vi "Initialize.vi"(8 "error in (no error)":errorcluster, 9 "Reset? (T: Yes)":bool=TRUE, 10 "ID Query? (T: Yes)":bool=TRUE, 11 "VISA resource name":refnum<visa-resource-name>) -> (0 "error out":errorcluster, 3 "VISA resource name out":refnum<visa-resource-name>)   [LabVIEW 2022 SP3, in "Agilent ENA Series.lvlib"]
doc: "Establishes communication with the instrument and optionally performs an instrument identification query and/or an instrument reset. It also places the instrument in a default state needed for other instrument driver operations. Therefore, call this VI before calling other instrument driver VIs for this instrument. Generally, you need to call the <B>Initialize VI</B> only once at the beginning of an application.\n\n<b>Note:</b>\nE5080A model support enabled by configuring the Emulation Mode \nSystem -> System Setting -> Code Emulation -> 5071"
uses:
  Agilent ENA Series.lvlib
  <vilib>/regexp/Match Regular Expression.xnode
panel:
  # "(c) 2005-2021 National Instruments.  ALL RIGHTS RESERVED."
  # "Note:\nE5080A, E5080B model support enabled by configuring the Emulation Mode \nSystem -> System Setting -> Code Emulation -> 5071"
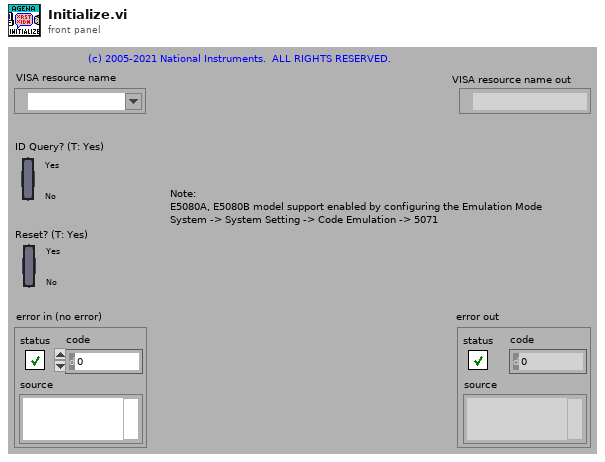
[diagram p1: front panel]
types:
  T1 = cluster{"Status":bool, "Code":i32, "Source (VI Name)":string}
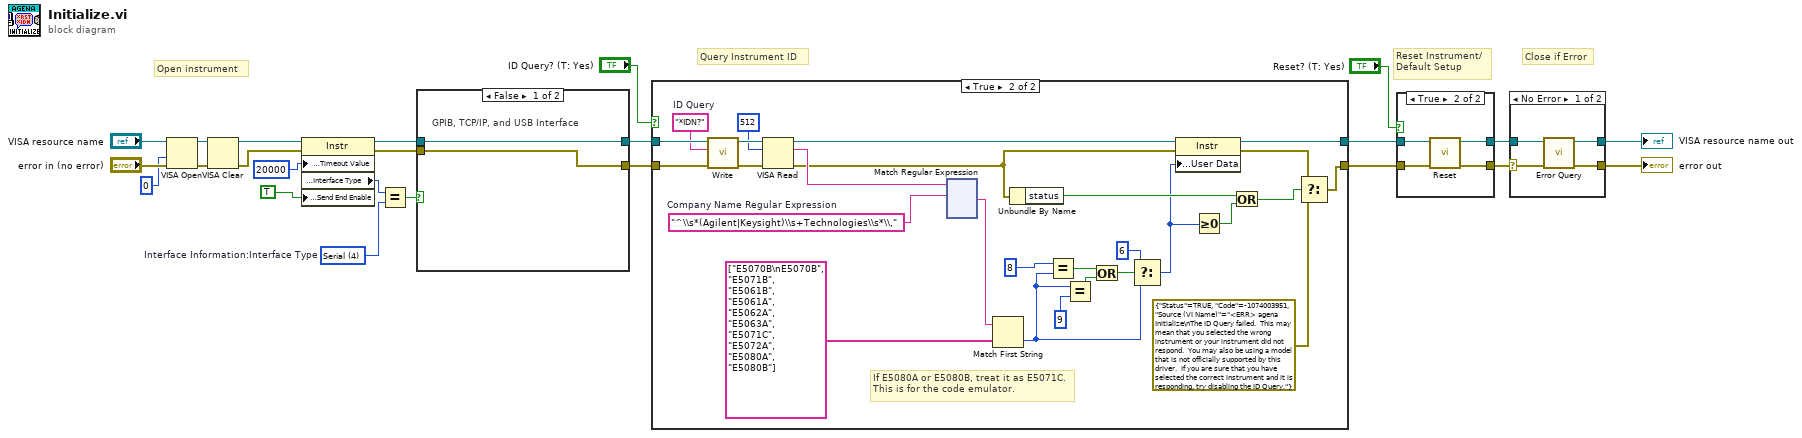
[diagram p0: block diagram]
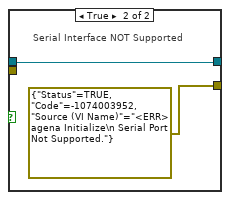
[diagram p2: hidden frame]
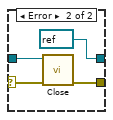
[diagram p3: hidden frame]
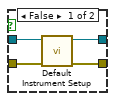
[diagram p4: hidden frame]
diagram:
  w13 = u16 4 items=["GPIB"=1, "VXI"=2, "GPIB-VXI"=3, "Serial"=4, "PXI"=5, "TCPIP"=6, "USB"=7]  # Interface Information:Interface Type
  # "Close if Error"
  # "Query Instrument ID"
  # "Reset Instrument/\nDefault Setup"
  # "Open instrument"
  n1 = VISA Open(access mode=u32 0, error in (no error)="error in (no error)", VISA resource name="VISA resource name") -> (VISA resource name=w3:refnum<visa-resource-name>, error out=w4:errorcluster)  [unwired: 2 in]
  n2 = VISA Clear(VISA resource name=w3, error in (no error)=w4) -> (VISA resource name out=w2:refnum<visa-resource-name>, error out=w1:errorcluster)
  n3 = property class="Instr"(reference=w2, error in=w1, "General Settings:Timeout Value"=u32 20000, "Message Based Settings:Send End Enable"=TRUE) -> (reference out=w16:refnum<visa-resource-name>, error out=w15:errorcluster, "Interface Information:Interface Type"=w18:u16)
  n4 = Equal?(x=w18, y=w13) -> (x = y?=w14:bool)
  n5 = case shown="False" w14 {
    tunnel: [w26 w28] -> w6
    tunnel: [w25 T1 {"Status"=TRUE, "Code"=-1074003952, "Source (VI Name)"="<ERR> agena Initialize\n Serial Port Not Supported."}] -> w5
    tunnel: w16 -> [w26 w28]
    tunnel: w15 -> [w25 _]
    frame False {
      # "GPIB, TCP/IP, and USB Interface"
    }
    frame True {
      # "Serial Interface NOT Supported"
    }
  }
  n6 = case shown="True" "ID Query? (T: Yes)" {
    tunnel: [w29 w57] -> w23
    tunnel: [w30 w43] -> w24
    tunnel: w6 -> [w30 w55]
    tunnel: w5 -> [w29 w56]
    frame False {
    }
    frame True {
      w40 = "^\\s*(Agilent|Keysight)\\s+Technologies\\s*\\,"  # Company Name Regular Expression
      w48 = "*IDN?"  # ID Query
      # "If E5080A or E5080B, treat it as E5071C.\nThis is for the code emulator."
      n7 = call "Write.vi"("error in (no error)"=w56, "String ()"=w48, "VISA resource name"=w55) -> ("error out"=w52:errorcluster, "VISA resource name out"=w53:refnum<visa-resource-name>)  [unwired: 6 in, 1 out]
      n8 = VISA Read(VISA resource name=w53, byte count=u32 512, error in (no error)=w52) -> (VISA resource name out=w44:refnum<visa-resource-name>, read buffer=w46:string, error out=w42:errorcluster)  [unwired: 1 out]
      n9 = xnode "Match Regular Expression"("input string"=w46, "regular expression"=w40) -> ("after match"=w39:string)  [unwired: 4 in, 4 out]
      n10 = Match First String(2:string[] ["E5070B\nE5070B", "E5071B", "E5061B", "E5061A", "E5062A", "E5063A", "E5071C", "E5072A", "E5080A", "E5080B"] ("string array"), 3:w39) -> (0:w35:i32)  [unwired: 1 out]
      n11 = Unbundle By Name(w42) -> ("status"=w50:bool)
      n12 = Equal?(x=8, y=w35) -> (x = y?=w33:bool)
      n13 = Equal?(x=w35, y=9) -> (x = y?=w32:bool)
      n14 = Or(x=w33, y=w32) -> (x .or. y?=w31:bool)
      n15 = Select(t=6, s=w31, f=w35) -> (s? t:f=w36:i32)
      n16 = property on="Property Node" class="Instr"(reference=w44, error in=w42, "General Settings:User Data"=w36) -> (reference out=w43:refnum<visa-resource-name>, error out=w41:errorcluster)
      n17 = Greater Or Equal To 0?(x=w36) -> (x >= 0?=w54:bool)
      n18 = Or(x=w50, y=w54) -> (x .or. y?=w51:bool)
      n19 = Select(t=w41, s=w51, f=T1 {"Status"=TRUE, "Code"=-1074003951, "Source (VI Name)"="<ERR> agena Initialize\nThe ID Query failed.  This may mean that you selected the wrong instrument or your instrument did not respond.  You may also be using a model that is not officially supported by this driver.  If you are sure that you have selected the correct instrument and it is responding, try disabling the ID Query."}) -> (s? t:f=w57:T1)
    }
  }
  n20 = case shown="True" "Reset? (T: Yes)" {
    tunnel: w23 -> [w177 w179]
    tunnel: [w176 w182] -> w8
    tunnel: w24 -> [w178 w180]
    tunnel: [w175 w181] -> w9
    frame False {
      n21 = call "Default Instrument Setup.vi"("error in (no error)"=w177, "VISA resource name"=w178) -> ("error out"=w176:errorcluster, "VISA resource name out"=w175:refnum<visa-resource-name>)  [unwired: 8 in]
    }
    frame True {
      n22 = call "Reset.vi"("error in (no error)"=w179, "VISA resource name"=w180) -> ("error out"=w182:errorcluster, "VISA resource name out"=w181:refnum<visa-resource-name>)  [unwired: 8 in]
    }
  }
  n23 = case shown="No Error" w8 {
    selector: w8 -> [w184 w188]
    tunnel: w9 -> [w183 w189]
    tunnel: [w186 refnum<visa-resource-name> refnum ("VISA resource name out")] -> w11
    tunnel: [w185 w190] -> w10
    frame No Error {
      n24 = call "Error Query.vi"("error in (no error)"=w184, "VISA resource name"=w183) -> ("error out"=w185:errorcluster, "VISA resource name out"=w186:refnum<visa-resource-name>)  [unwired: 6 in, 2 out]
    }
    frame Error {
      n25 = call "Close.vi"("error in (no error)"=w188, "VISA resource name"=w189) -> ("error out"=w190:errorcluster)  [unwired: 9 in]
    }
  }
  "VISA resource name out" <- w11
  "error out" <- w10
